vi "swerveBegin.vi"(0 "center gravity (x)":dbl, 1 "center gravity (y)":dbl, 2 "robot width (x)":dbl, 3 "robot length (y)":dbl) -> ()   [LabVIEW 2019]
uses:
  swerveData.vi
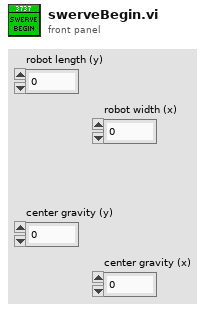
[diagram p1: front panel]
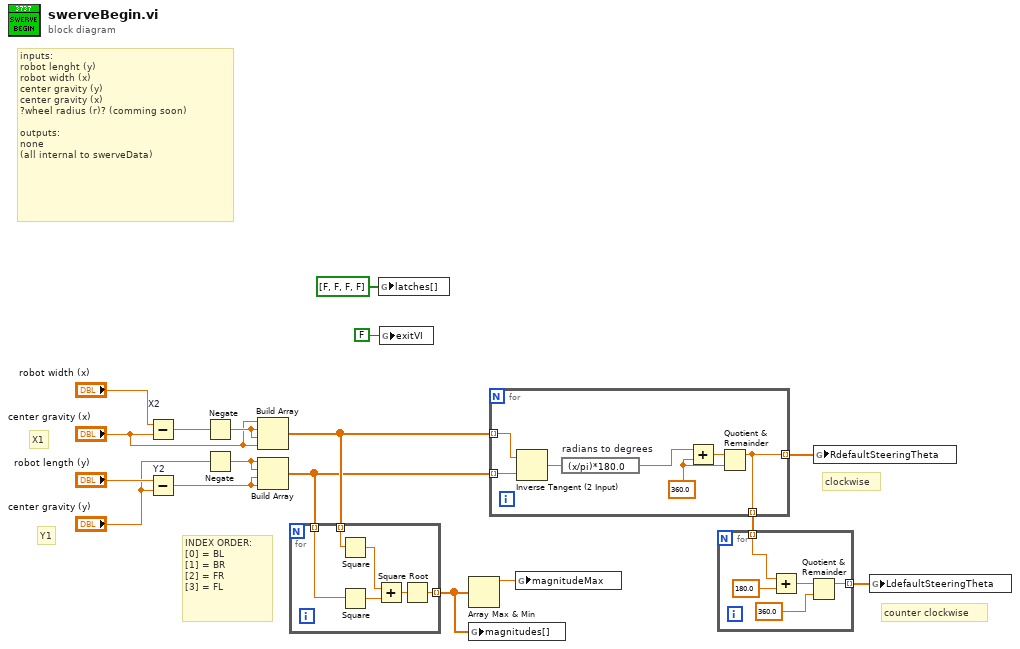
[diagram p0: block diagram]
diagram:
  # "INDEX ORDER:\n[0] = BL\n[1] = BR\n[2] = FR\n[3] = FL"
  # "counter clockwise"
  # "clockwise"
  # "X1"
  # "Y1"
  # "inputs:\nrobot lenght (y)\nrobot width (x)\ncenter gravity (y)\ncenter gravity (x)\n?wheel radius (r)? (comming soon)\n\noutputs:\nnone\n(all internal to swerveData)"
  n1 = Subtract "X2"(x="robot width (x)", y="center gravity (x)") -> (x-y=w12:dbl)
  n2 = Subtract "Y2"(x="robot length (y)", y="center gravity (y)") -> (x-y=w13:dbl)
  n3 = Negate(x=w12) -> (-x=w16:dbl)
  n4 = Negate(x="center gravity (y)") -> (-x=w17:dbl)
  n5 = Build Array("center gravity (x)", w16, w16, "center gravity (x)") -> (w11:dbl[])
  n6 = Build Array(w17, w17, w13, w13) -> (w10:dbl[])
  n7 = for {
    tunnel: w11 -> [w20] mode=indexing
    tunnel: w10 -> [w19] mode=indexing
    tunnel: [w18] -> w8 mode=indexing
    n8 = Square(x=w20) -> (x^2=w21:dbl)
    n9 = Square(x=w19) -> (x^2=w22:dbl)
    n10 = Add(x=w21, y=w22) -> (x+y=w23:dbl)
    n11 = Square Root(x=w23) -> (sqrt(x)=w18:dbl)
  }
  n12 = global write "swerveData.vi" "latches[]"(bool[] [FALSE, FALSE, FALSE, FALSE] ("latches[]")) -> ()
  n13 = global write "swerveData.vi" "exitVI"(FALSE ("exitVI")) -> ()
  n14 = Array Max & Min(array=w8) -> (max value=w9:dbl)  [unwired: 3 out]
  n15 = global write "swerveData.vi" "magnitudes[]"(w8) -> ()
  n16 = for {
    tunnel: w11 -> [w29] mode=indexing
    tunnel: w10 -> [w28] mode=indexing
    tunnel: [w26] -> w14 mode=indexing
    tunnel: [w26] -> w15 mode=indexing
    w24 = 360.0 ("x")
    n17 = Inverse Tangent (2 Input)(1:w28, 2:w29) -> (0:w30:dbl)
    n18 = expression code="(x/pi)*180.0" "radians to degrees"(w30) -> (w25:dbl)
    n19 = Add(x=w25, y=w24) -> (x+y=w27:dbl)
    n20 = Quotient & Remainder(x=w27, y=w24) -> (x-y*floor(x/y)=w26:dbl)  [unwired: 1 out]
  }
  n21 = global write "swerveData.vi" "magnitudeMax"(w9) -> ()
  n22 = for {
    tunnel: w15 -> [w34] mode=indexing
    tunnel: [w31] -> w7 mode=indexing
    n23 = Add(x=w34, y=180.0) -> (x+y=w33:dbl)
    n24 = Quotient & Remainder(x=w33, y=360.0 ("x")) -> (x-y*floor(x/y)=w31:dbl)  [unwired: 1 out]
  }
  n25 = global write "swerveData.vi" "RdefaultSteeringTheta"(w14) -> ()
  n26 = global write "swerveData.vi" "LdefaultSteeringTheta"(w7) -> ()
